vi "Test Return Test Case Result for Parametrized Case When Running Filtered.vi"(11 "Test Case In":refnum<class "Parameterized Test Case Test.lvclass">) -> (0 "error out":errorcluster, 3 "Test Case Out":refnum<class "Parameterized Test Case Test.lvclass">)   [LabVIEW 2020, in "Parameterized Test Case Test.lvclass"]
uses:
  Parameterized Test Case Test.lvclass
  C:/Program Files (x86)/National Instruments/LabVIEW 2020/vi.lib/Astemes/LUnit/Test Case.lvclass
  <vilib>/Astemes/LUnit/Test Case.lvclass/Test Case.ctl
  399136ac-e113-4bca-be3a-8dde4e32c814.vi
  <vilib>/Astemes/LUnit/Palette/Pass If.vi
  <vilib>/Astemes/LUnit/Core/LUnit Test Case/Private/Append Fail Result.vi
  <vilib>/Astemes/LUnit/Core/LUnit Test Case/Private/Append Pass Result.vi
  <vilib>/Astemes/LUnit/Core/LUnit Test Case/Private/Run In UI.vi
  <vilib>/Utility/error.llb/Clear Errors.vi
  source/Parameterized Test Case/Parameterized Test Case.lvclass
  <vilib>/Astemes/LUnit/Test Suite.lvclass
panel:
  out "List of Runnables 2":string[](array[string])
  out "List of Runnables":string[](array[string])
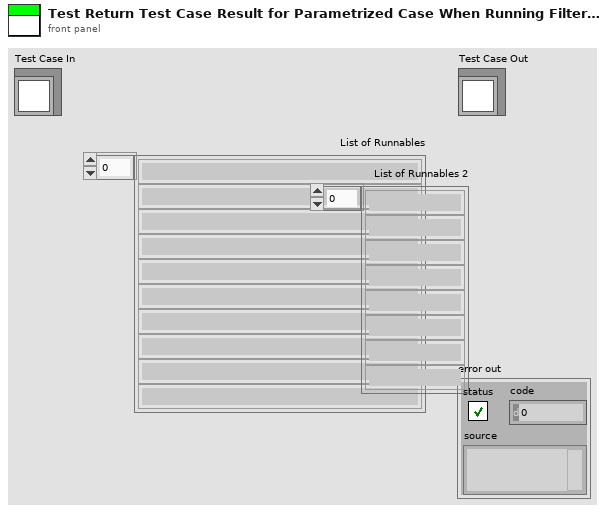
[diagram p1: front panel]
types:
  T1 = cluster{"Name":string, "Description":string, "Status":enum16{"", "Passed", "Failed", "Error", "Skipped", "Setup Error", "Broken", "Teardown Error"}, "Result Type":enum16{"Test Case", "Test Suite", "Test Run", "Pass", "Fail", "Skip", "Pass if", "Fail if", "Pass if Error", "Fail if Error", "Pass if Equal", "Fail if Equal"}, "Execution Time":dbl, "Data":cluster{"Expected":variant, "Actual":variant, "Delta":variant}}[]
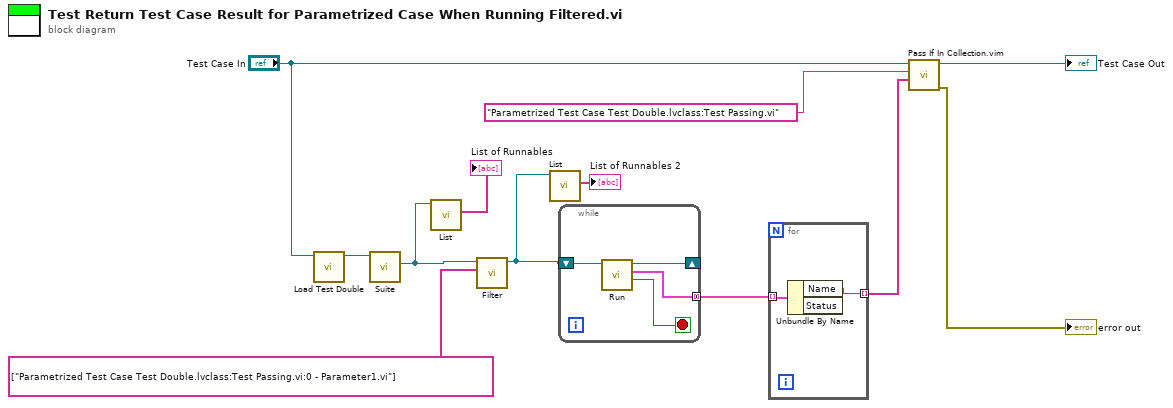
[diagram p0: block diagram]
diagram:
  n1 = call "Load Test Double.vi"("Parameterized Test Case Test in"="Test Case In") -> ("Parameterized Test Case out"=w6:refnum<class "Parameterized Test Case.lvclass">)  [unwired: 9 in, 1 out]
  n2 = call-dynamic "Suite.vi"("Parameterized Test Case In"=w6) -> ("LUnit Test Suite Out"=w4:refnum<class "Test Suite.lvclass">)  [unwired: 8 in, 2 out]
  n3 = call <vilib>:"List.vi"("LUnit Test Suite In"=w4) -> ("List of Runnables"=→"List of Runnables":string[])  [unwired: 9 in, 1 out]
  n4 = call <vilib>:"Filter.vi"("Selected Runnables"=string[] ["Parametrized Test Case Test Double.lvclass:Test Passing.vi:0 - Parameter1.vi"], "LUnit Test Suite In"=w4) -> ("LUnit Test Suite Out"=w3:refnum<class "Test Suite.lvclass">)  [unwired: 8 in, 1 out]
  n5 = call <vilib>:"List.vi"("LUnit Test Suite In"=w3) -> ("List of Runnables"=→"List of Runnables 2":string[])  [unwired: 9 in, 1 out]
  n6 = while {
    tunnel: [w16] -> w9 mode=concatenating
    shift-right: [w15] -> _
    shift-left: w3 -> [w13]
    stop <- w14 stop-if-true
    n7 = call-dynamic "Run.vi"("LUnit Test Suite In"=w13) -> ("Done?"=w14:bool, "Results"=w16:T1, "LUnit Test Suite In 2"=w15:refnum<class "Test Suite.lvclass">)  [unwired: 7 in, 1 out]
  }
  n8 = for {
    tunnel: w9 -> [w18] mode=indexing
    tunnel: [w17] -> w8 mode=indexing
    n9 = Unbundle By Name(w18) -> ("Name"=w17:string)  [unwired: 1 out]
  }
  n10 = call "Pass If In Collection.vim"("Collection"=w8, "Expected Element"="Parametrized Test Case Test Double.lvclass:Test Passing.vi" ("String"), "LUnit Test Case In"="Test Case In") -> ("error out"=→"error out":errorcluster, "LUnit Test Case Out"=→"Test Case Out":refnum<class "Parameterized Test Case Test.lvclass">)  [unwired: 7 in]
